vi "8bit sync-Disable ctrls.vi"(8 "error in (no error)":errorcluster, 10 "Disabled":T1(ring)) -> (0 "error out":errorcluster)   [LabVIEW 2017]
uses:
  Globals/gl_8-bit montage window ctrl refs.vi
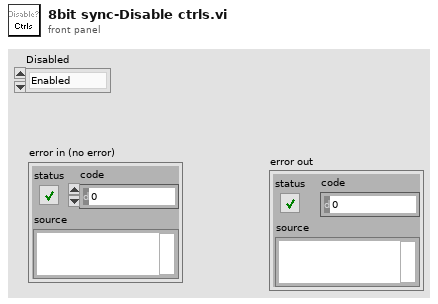
[diagram p1: front panel]
types:
  T1 = enum8{"Enabled", "Disabled", "Disabled and Grayed Out"}
  T2 = typedef "8-bit video export window ctrl refs.ctl" = cluster{"This VI":refnum<vi>, "Add speed data":refnum<vi>, "Add camera videos":refnum<vi>, "Stop button":refnum<vi>, "Camera Video Adjustments":refnum<vi>, "Microscope Image Adjustments":refnum<vi>, "Execute":refnum<vi>, "Codec":refnum<vi>, "Channel to load":refnum<vi>, "Speed graph behaviour":refnum<vi>, "Include speed graph":refnum<vi>, "Number of rows to generate":refnum<vi>, "Path":refnum<vi>}
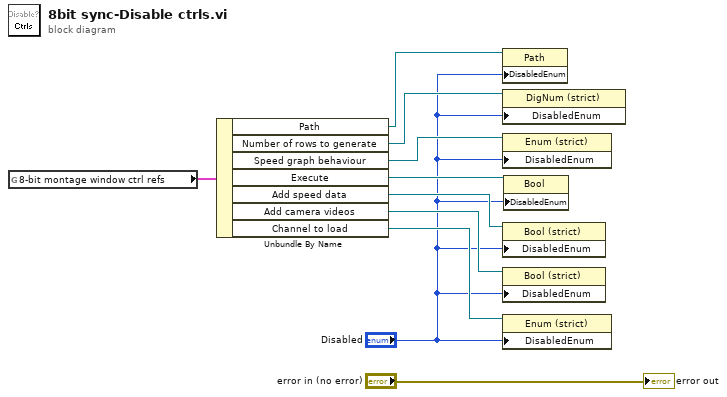
[diagram p0: block diagram]
diagram:
  n1 = global read "gl_8-bit montage window ctrl refs.vi" "8-bit montage window ctrl refs"() -> (w10:T2)
  n2 = Unbundle By Name(w10) -> ("Path"=w2:refnum<vi>, "Number of rows to generate"=w3:refnum<vi>, "Speed graph behaviour"=w4:refnum<vi>, "Execute"=w9:refnum<vi>, "Add speed data"=w8:refnum<vi>, "Add camera videos"=w7:refnum<vi>, "Channel to load"=w6:refnum<vi>)
  n3 = property on="Property Node" class="Path"(reference=w2, "DisabledEnum"="Disabled") -> ()  [unwired: 1 in, 2 out]
  n4 = property on="Property Node" class="DigNum (strict)"(reference=w3, "DisabledEnum"="Disabled") -> ()  [unwired: 1 in, 2 out]
  n5 = property on="Property Node" class="Enum (strict)"(reference=w4, "DisabledEnum"="Disabled") -> ()  [unwired: 1 in, 2 out]
  n6 = property on="Property Node" class="Bool (strict)"(reference=w8, "DisabledEnum"="Disabled") -> ()  [unwired: 1 in, 2 out]
  n7 = property on="Property Node" class="Bool (strict)"(reference=w7, "DisabledEnum"="Disabled") -> ()  [unwired: 1 in, 2 out]
  n8 = property on="Property Node" class="Enum (strict)"(reference=w6, "DisabledEnum"="Disabled") -> ()  [unwired: 1 in, 2 out]
  n9 = property on="Property Node" class="Bool"(reference=w9, "DisabledEnum"="Disabled") -> ()  [unwired: 1 in, 2 out]
  "error out" <- "error in (no error)"
